vi "Timestamp.vi"(11 "TimestampSettings":T1={"TimeSource"="5MHz", "TimeRegister"="Time", "IterationsPerMicrosecond"=0, "UpdateFIFO"="TimestampUpdate", "HealthAndStatusFIFO"="TimestampUpdate", "HealthAndStatusAddress"=0, "IterationsPerHealthAndStatusUpdate"=0}) -> ()   [LabVIEW 2016, in "FPGATimestamp.lvlib"]
uses:
  FPGATimestamp.lvlib
  DataTypes/TimestampSettings.ctl
  <vilib>/Platform/TimedLoop/XDataNode/timing_clust.ctl
  <vilib>/Platform/TimedLoop/XDataNode/nitl_modes.ctl
  <vilib>/Platform/TimedLoop/XDataNode/wakeup.ctl
  Common_FPGA_HealthAndStatus/DataTypes/HealthAndStatusUpdateMode.ctl
  <vilib>/rvi/Emulation/niFpgaSctlEmulationGetInTimedLoop.vi
  <vilib>/rvi/Emulation/niFpgaEmulationReportErrorSimple.vi
  <vilib>/rvi/Emulation/niFpgaGetClockAttributes.vi
  <vilib>/rvi/Emulation/niFpgaCriticalErrorInLSC.vi
  <vilib>/rvi/DataTransferAndStorage/Container/Common/niFpgaContainerExecOnDevCompGetState.vi
  <vilib>/rvi/Emulation/niFpgaEmulationIsFPGAContextNoSignature.vi
  <vilib>/rvi/DataTransferAndStorage/Container/Common/niFpgaContainerGetUniqueNameForEmu.vi
  <vilib>/rvi/Memory/Memory_Emulation/niFpgaMemoryEmulationCacheClearOnFirstRun.vi
  <vilib>/rvi/Memory/Memory_Emulation/nirvimemoryEmulationManagerCache_MakeExclusive.vi
  <vilib>/rvi/Memory/Memory_Emulation/niFpgaMemoryEmulationValidateCache.vi
  <vilib>/rvi/Memory/Memory_Emulation/nirvimemoryEmulationManagerCache_InsertValue.vi
  <vilib>/Utility/error.llb/Clear Errors.vi
  <vilib>/rvi/Memory/Memory_Emulation/nirvimemoryEmulationManagerCache_ReleaseExclusive.vi
  <vilib>/rvi/Memory/Memory_Emulation/nirvimemoryEmulationManagerCache_GetValue.vi
  <vilib>/rvi/Memory/Memory_Emulation/nirvimemoryEmulationManagerCache_SetValue.vi
  <vilib>/rvi/Emulation/niFpgaProcessEmulError.vi
  <vilib>/rvi/errors/niFpgaSetErrorForExecOnDevCompSimple.vi
  <vilib>/rvi/eio/common/nirviEmuReportErrorAndStop.vi
  <vilib>/rvi/FIFO/Fifo_Resource/nirvififoEmulationSetSize.vi
  <vilib>/rvi/FIFO/Fifo_Resource/nirviFifoEmulationQueueMgr.vi
  <instcachedir>/0/nirviFifoEmulationQueueMgr_E5CAEC123FF24DC58D834DCA3CDAA9B5.lvgen/nirviFifoEmulationQueueMgr_E5CAEC123FF24DC58D834DCA3CDAA9B5_007.vi
  <vilib>/rvi/FIFO/Fifo_Resource/nirvififoEmulationDetermineInputValidOut.vi
  <vilib>/rvi/FIFO/Fifo_Resource/nirvififoEmulationCreateLock.vi
  <vilib>/rvi/FIFO/Fifo_Resource/nirvififoEmulationObtainLock.vi
  <vilib>/rvi/FIFO/Fifo_Resource/nirvififoEmulationReleaseLock.vi
  <vilib>/rvi/occurrence/nirviWaitOnOccurrenceBase.vi
  <vilib>/rvi/errors/nirviReportUnexpectedCaseInternalError.vi
  <vilib>/rvi/errors/nirviReportUnexpectedCaseInternalError (U32).vi
  <vilib>/rvi/interface/RandomDataEmulation/niFpgaRandomDataHandleErrors.vi
  <vilib>/Platform/TimedLoop/XDataNode/XDataNode.xnode
  <vilib>/rvi/DataTransferAndStorage/Container/XNode/niFpgaContainer.xnode
  <vilib>/rvi/DataTransferAndStorage/Register/Emulation/niFpgaRegisterEmulationRefIn.vi
  <vilib>/rvi/FIFO/Fifo_Resource/niFpgaFifoEmulationRefIn.vi
  <vilib>/Platform/TimedLoop/XDataNode/XDNodeRunTimeDep.lvlib
  Common_FPGA_HealthAndStatus/FPGAHealthAndStatus.lvlib
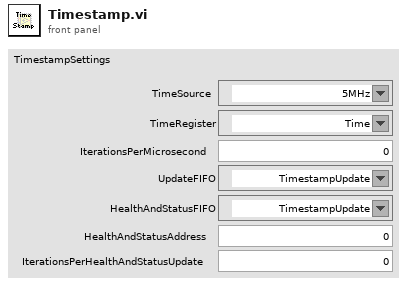
[diagram p1: front panel]
types:
  T1 = typedef "FPGATimestamp.lvlib/TimestampSettings.ctl" = cluster{"TimeSource":refnum<k21>, "TimeRegister":refnum<k21>, "IterationsPerMicrosecond":i16, "UpdateFIFO":refnum<k21>, "HealthAndStatusFIFO":refnum<k21>, "HealthAndStatusAddress":i16, "IterationsPerHealthAndStatusUpdate":i16}
  T2 = typedef "XDNodeRunTimeDep.lvlib/timing_clust.ctl" = cluster{"Expected End [f-1]":u64, "Actual End [f-1]":u64, "Finished Late? [f-1]":bool, "Expected End [i-1]":u64, "Actual End [i-1]":u64, "Finished Late? [i-1]":bool, "Expected Start [i]":u64, "Actual Start [i]":u64, "Expected Start [f]":u64, "Actual Start [f]":u64, "Source Name":string, "Structure Name":string, "Period":i64, "Deadline":i64, "Offset":i64, "Start":i64, "Priority":i32, "Timeout":i32, "Mode":T3, "Wakeup Reason":T4, "Error":errorcluster, "Source Type":string, "Secondary Source Type":string, "Global End Time":u64, "Global Start Time":u64, "Frame Duration":u64, "Iteration Duration":u64, "Assigned CPU":i32, "I/O Scan Engine Mode":u32}
  T3 = typedef "XDNodeRunTimeDep.lvlib/nitl_modes.ctl" = enum32{"No Change", "Process missed periods, maintain original phase", "Discard missed periods, maintain original phase", "Process missed periods, ignore original phase", "Discard missed periods, ignore original phase"}
  T4 = typedef "XDNodeRunTimeDep.lvlib/wakeup.ctl" = enum32{"Normal", "Aborted", "Asynchronous wakeup", "Timing source error", "Timed loop error", "Timeout"}
  T5 = typedef "FPGAHealthAndStatus.lvlib/HealthAndStatusUpdateMode.ctl" = enum8{"NOP", "Set", "Add", "Subtract", "Or"}
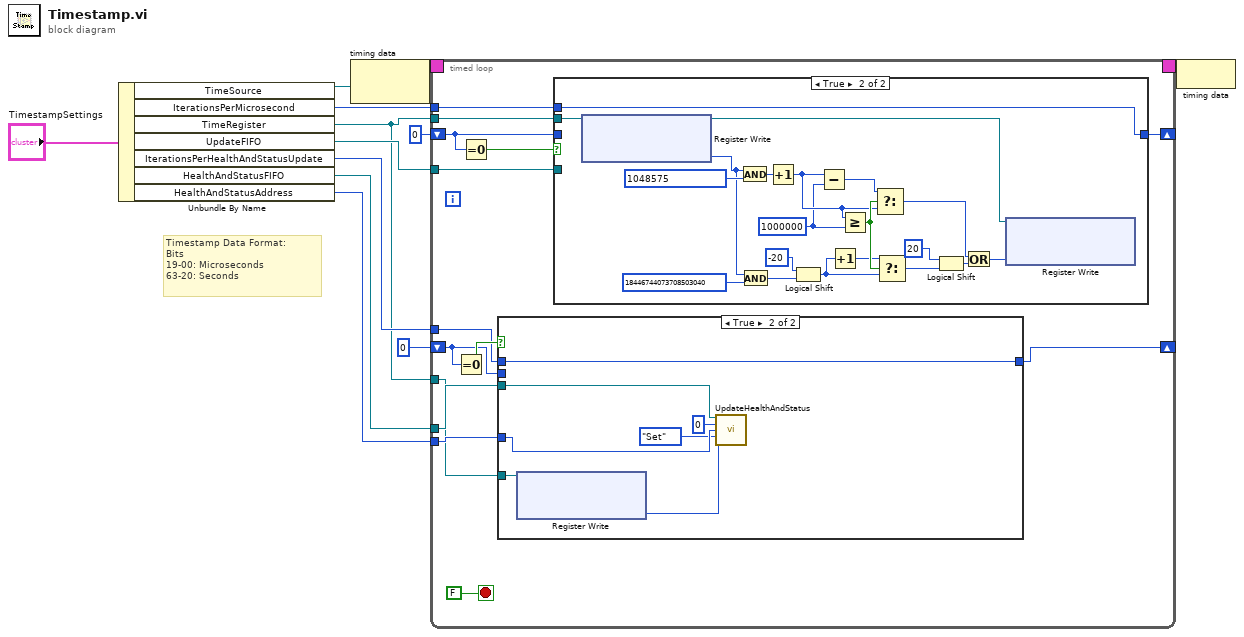
[diagram p0: block diagram]
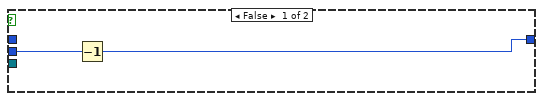
[diagram p2: hidden frame]
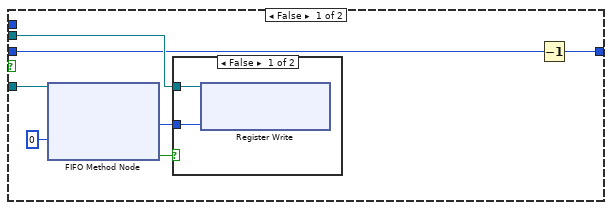
[diagram p3: hidden frame]
diagram:
  # "Timestamp Data Format:\nBits\n19-00: Microseconds\n63-20: Seconds"
  n1 = Unbundle By Name("TimestampSettings") -> ("TimeSource"=w9:refnum<k21>, "IterationsPerMicrosecond"=w8:i16, "TimeRegister"=w1:refnum<k21>, "UpdateFIFO"=w7:refnum<k21>, "IterationsPerHealthAndStatusUpdate"=w5:i16, "HealthAndStatusFIFO"=w4:refnum<k21>, "HealthAndStatusAddress"=w3:i16)
  n2 = node-c288 ("Input Node")(w9) -> (w12:T2)
  n3 = timed-loop {
    timing: w12 -> [_]
    timing-out: [_] -> w11
    shift-right: [w24] -> _
    shift-left: i16 0 -> [w25]
    tunnel: w1 -> [w22]
    tunnel: w8 -> [w21]
    tunnel: w7 -> [w20]
    shift-right: [w18] -> _
    shift-left: i16 0 -> [w16]
    tunnel: w5 -> [w17]
    tunnel: w4 -> [w15]
    tunnel: w3 -> [w14]
    tunnel: w1 -> [w13]
    stop <- FALSE stop-if-true
    n4 = Equal To 0?(x=w16) -> (x = 0?=w19:bool)
    n5 = Equal To 0?(x=w25) -> (x = 0?=w26:bool)
    n6 = case shown="True" w19 {
      tunnel: w16 -> [w28 _]
      tunnel: [w27 w35] -> w18
      tunnel: w17 -> [_ w35]
      tunnel: w15 -> [_ w31]
      tunnel: w14 -> [_ w32]
      tunnel: w13 -> [_ w34]
      frame False {
        n7 = Decrement(x=w28) -> (x-1=w27:i16)
      }
      frame True {
        n8 = xnode ("Register Write")("Register In"=w34) -> ("Data"=w33:u64)  [unwired: 1 out]
        n9 = call "UpdateHealthAndStatus.vi"("InternalHealthAndStatusFIFO"=w31, "AddressOffset"=u32 0, "BaseAddress"=w32, "HealthAndStatusUpdateMode"=HealthAndStatusUpdateMode."Set", "Data"=w33) -> ()  [unwired: 11 in]
      }
    }
    n10 = case shown="True" w26 {
      tunnel: w25 -> [w37 _]
      tunnel: [w36 w49] -> w24
      tunnel: w22 -> [w38 w47]
      tunnel: w21 -> [_ w49]
      tunnel: w20 -> [w41 _]
      frame False {
        n11 = xnode ("FIFO Method Node")("Timeout"=0, "FIFO In"=w41) -> ("Element"=w39:u64, "Timed Out?"=w40:bool)  [unwired: 1 out]
        n12 = case shown="False" w40 {
          tunnel: w39 -> [w43 _]
          tunnel: w38 -> [w44 _]
          frame False {
            n13 = xnode ("Register Write")("Data"=w43, "Register In"=w44) -> ()  [unwired: 1 out]
          }
          frame True {
          }
        }
        n14 = Decrement(x=w37) -> (x-1=w36:i16)
      }
      frame True {
        w50 = u64 1000000 ("y")
        n15 = xnode ("Register Write")("Register In"=w47) -> ("Data"=w45:u64, "Register Out"=w46:refnum<k21>)
        n16 = And(x=w45, y=u64 1048575) -> (x .and. y?=w63:u64)
        n17 = And(x=w45, y=u64 18446744073708503040) -> (x .and. y?=w61:u64)
        n18 = Increment(x=w63) -> (x+1=w57:u64)
        n19 = Logical Shift(y=i16 -20, x=w61) -> (x << y=w60:u64)
        n20 = Subtract(x=w57, y=w50) -> (x-y=w58:u64)
        n21 = Increment(x=w60) -> (x+1=w51:u64)
        n22 = Greater Or Equal?(x=w57, y=w50) -> (x >= y?=w59:bool)
        n23 = Select(t=w58, s=w59, f=w57) -> (s? t:f=w53:u64)
        n24 = Select(t=w51, s=w59, f=w60) -> (s? t:f=w56:u64)
        n25 = Logical Shift(y=i16 20, x=w56) -> (x << y=w52:u64)
        n26 = Or(x=w53, y=w52) -> (x .or. y?=w48:u64)
        n27 = xnode ("Register Write")("Data"=w48, "Register In"=w46) -> ()  [unwired: 1 out]
      }
    }
  }
  n28 = node-c288(w11) -> ()
